vi "USRP Sampling.vi"(3 "parameter":T1={"Method"=enum."Binary", "offset"=0, "threshold"=1.0, "step"=1.0}, 4 "SamplingTimes":i32=100, 5 "Wifi Channel":i32=3, 6 "device names":refnum<k15>="192.168.10.2") -> (0 "error out":errorcluster, 1 "output":dbl[][](array[numeric]), 2 "coerced carrier frequency":dbl=2421999999.997206 format="%#_6p")   [LabVIEW 2014]
uses:
  <instrlib>/niUSRP/niUSRP Fetch Rx Data (CDB Cluster).vi
panel:
  out "n":i32
  out "Waveform Graph":dbl[](graph)
  out "Iteration":i32
  out "Array":dbl[](array[numeric])
  in  "stop":bool
  in  "Tab Control":enum32{"USRP Setup", "Parameter"}(tab)
  in  "IQ rate":dbl=800000.0 format="%#_6p"
  in  "gain":dbl=10.0 format="%#_6f"
  out "coerced IQ rate":dbl=800000.0 format="%#_6p"
  out "coerced gain":dbl=10.0 format="%#_6f"
  in  "active antenna":string="RX2"
  out "Duration(s)":dbl
  in  "Moving\nAverage":bool=TRUE
  in  "Time Window(s)":dbl=0.01 format="%#_6p"
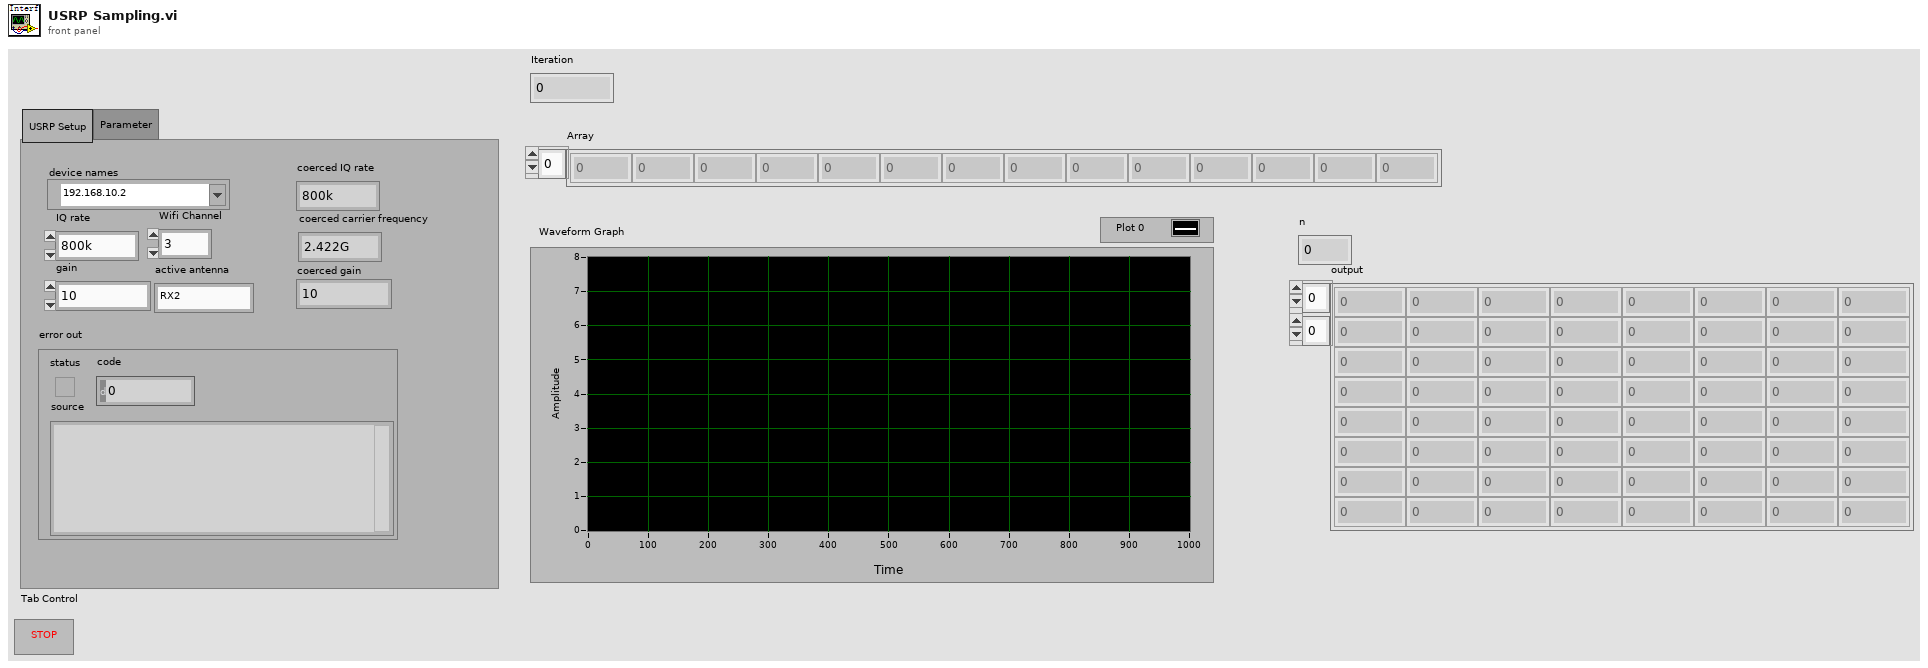
[diagram p1: front panel]
types:
  T1 = cluster{"Method":enum16{"Binary", "Uniform"}, "offset":i32, "threshold":dbl, "step":dbl}
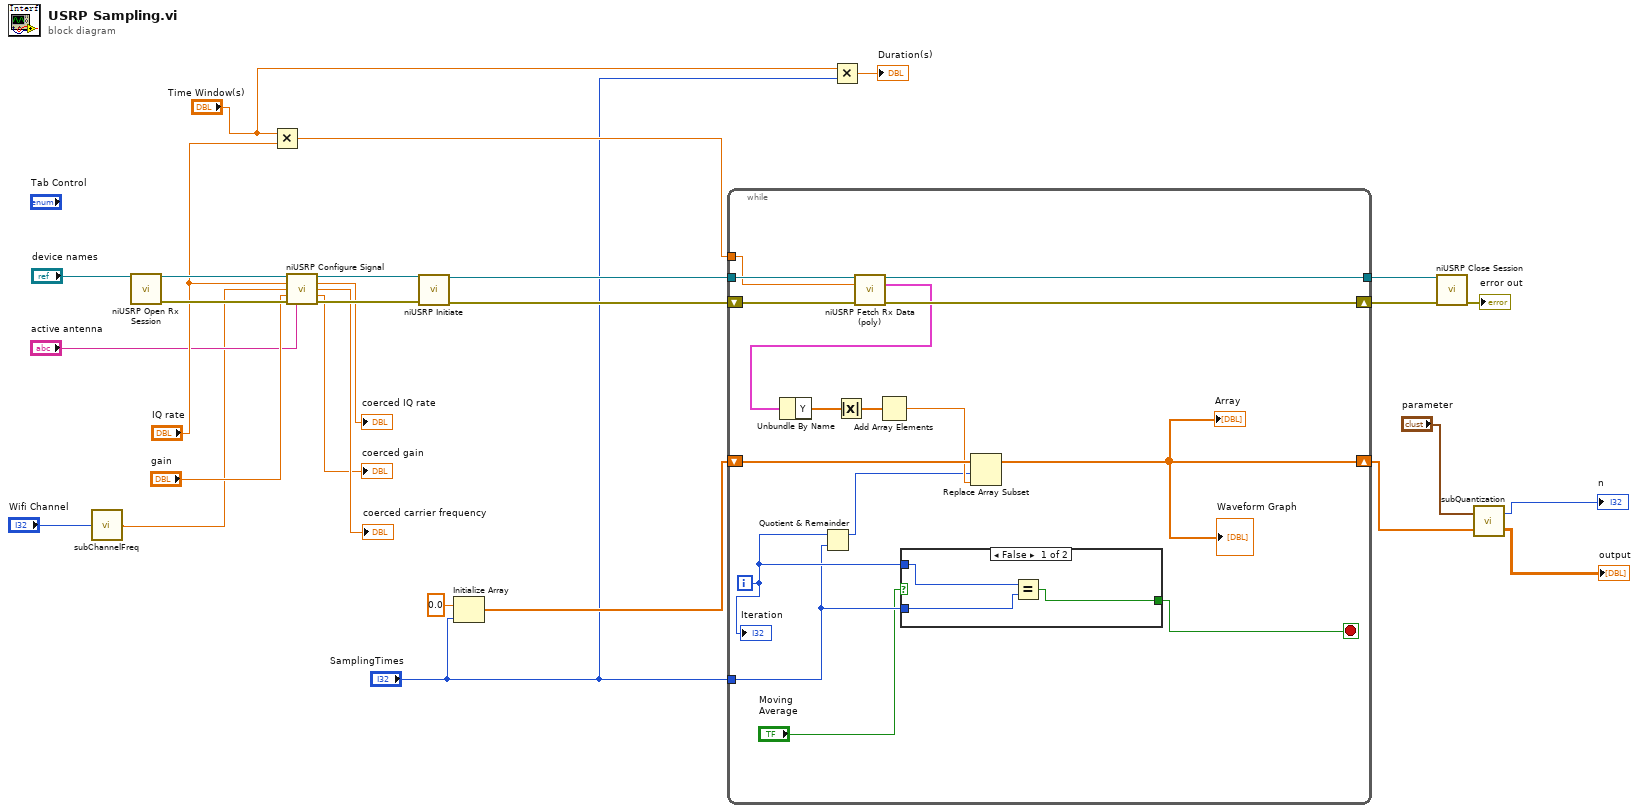
[diagram p0: block diagram]
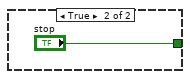
[diagram p2: hidden frame]
diagram:
  n1 = call "subChannelFreq.vi"("Channel"="Wifi Channel") -> ("Freq."=w5:dbl)
  n2 = call <instrlib>:"niUSRP Open Rx Session.vi"("device names"="device names") -> ("session handle out"=w26:refnum<k15>, "error out"=w27:errorcluster)  [unwired: 13 in]
  n3 = Multiply(x="Time Window(s)", y="IQ rate") -> (x*y=w10:dbl)
  n4 = call <instrlib>:"niUSRP Configure Signal.vi"("session handle"=w26, "IQ rate"="IQ rate", "carrier frequency"=w5, "gain"="gain", "error in (no error)"=w27, "active antenna"="active antenna") -> ("session handle out"=w25:refnum<k15>, "coerced IQ rate"=→"coerced IQ rate":dbl, "coerced carrier frequency"=→"coerced carrier frequency":dbl, "coerced gain"=→"coerced gain":dbl, "error out"=w24:errorcluster)  [unwired: 5 in]
  n5 = call <instrlib>:"niUSRP Initiate.vi"("session handle"=w25, "error in (no error)"=w24) -> ("session handle out"=w19:refnum<k15>, "error out"=w18:errorcluster)  [unwired: 12 in]
  n6 = Initialize Array(0.0 ("element"), "SamplingTimes") -> (w12:dbl[])
  n7 = while {
    tunnel: w19 -> [w44]
    tunnel: [w41] -> w16
    shift-right: [w42] -> w17
    shift-left: w18 -> [w43]
    shift-right: [w32] -> w3
    shift-left: w12 -> [w37]
    tunnel: "SamplingTimes" -> [w31]
    tunnel: w10 -> [w30]
    i -> [w33]
    stop <- w34 stop-if-true
    n8 = Quotient & Remainder(x=w33, y=w31) -> (x-y*floor(x/y)=w35:i32)  [unwired: 1 out]
    n9 = call-poly <instrlib>:"niUSRP Fetch Rx Data (poly).vi"("session handle"=w44, "number of samples"=w30, "error in (no error)"=w43) -> ("session handle out"=w41:refnum<k15>, "data"=w40:cluster{"t0":dbl, "dt":dbl, "Y":cdb[]}, "error out"=w42:errorcluster)  [unwired: 9 in, 1 out]
    n10 = Unbundle By Name(w40) -> ("Y"=w39:cdb[])
    n11 = Absolute Value(x=w39) -> (abs(x)=w38:dbl[])
    n12 = Add Array Elements(numeric array=w38) -> (sum=w36:dbl)
    n13 = case shown="False" "Moving\nAverage" {
      tunnel: [w45 "stop"] -> w34
      tunnel: w33 -> [w47 _]
      tunnel: w31 -> [w46 _]
      frame False {
        n14 = Equal?(x=w47, y=w46) -> (x = y?=w45:bool)
      }
      frame True {
      }
    }
    n15 = Replace Array Subset(array=w37, new element=w36, index=w35) -> (w32:dbl[])
    "Array" <- w32
    "Waveform Graph" <- w32
    "Iteration" <- w33
  }
  n16 = Multiply(x="Time Window(s)", y="SamplingTimes") -> (x*y=→"Duration(s)":dbl)
  n17 = call <instrlib>:"niUSRP Close Session.vi"("session handle"=w16, "error in (no error)"=w17) -> ("error out"=→"error out":errorcluster)  [unwired: 13 in]
  n18 = call "subQuantization.vi"("input"=w3, "parameter"="parameter") -> ("output"=→"output":dbl[][], "n"=→"n":i32)
